vi "create func files.vi"(11 "path":path) -> (2 "funtions.c":string, 3 "funtions.h":string)   [LabVIEW 2010]
uses:
  read_excel_values.llb/GetXL_CellValues_2D_String.vi
panel:
  out "error out":errorcluster
  # "Type: U8, I8, U16, I16, U32, I32, U64, I64, FLOAT"
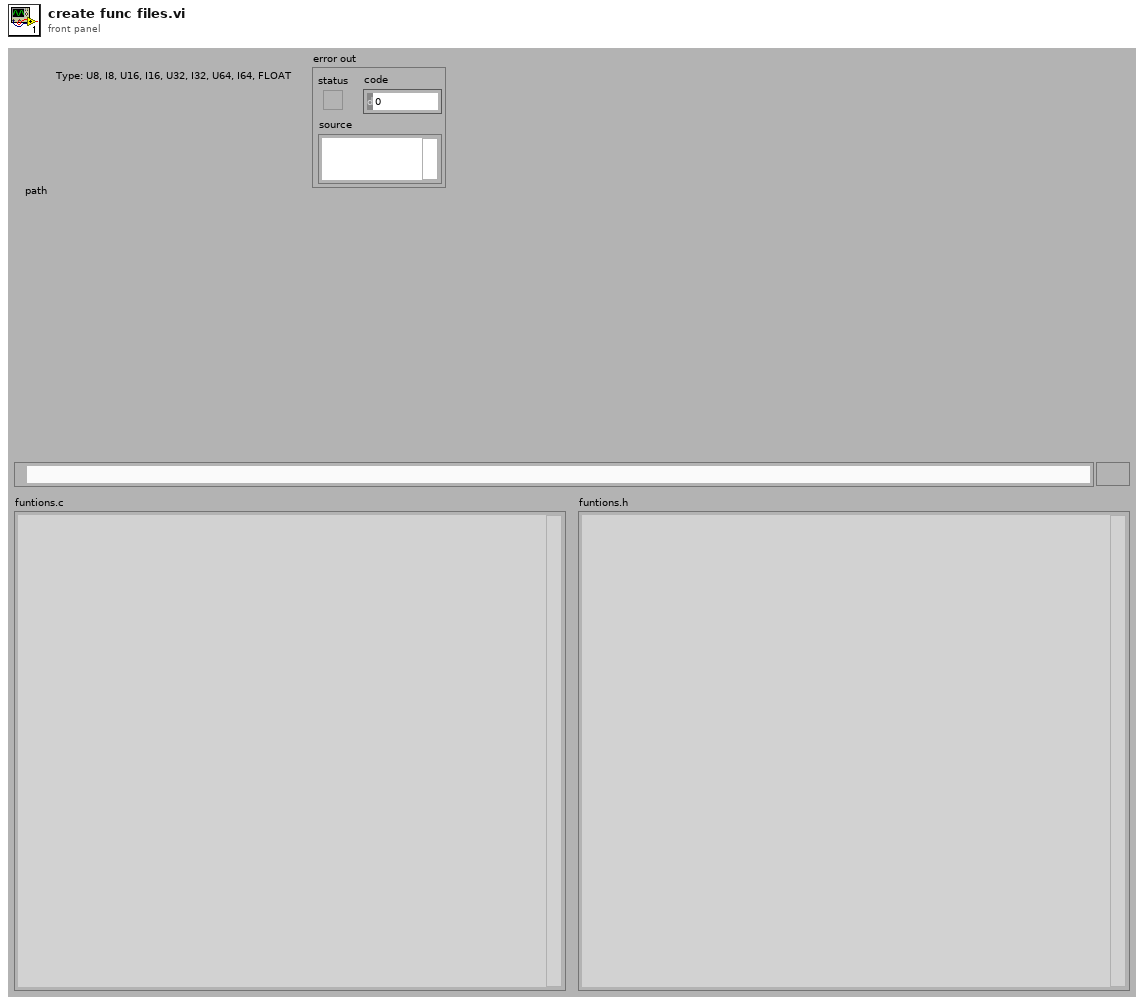
[diagram p1: front panel]
types:
  T1 = cluster{"Excel._Application":refnum<k7>, "Workbooks":refnum<k7>}
  T2 = cluster{"Excel._Application":refnum<k7>, "Workbooks":refnum<k7>, "Open":refnum<k7>}
  T3 = cluster{"Excel._Application":refnum<k7>, "Workbooks":refnum<k7>, "Open":refnum<k7>, "Worksheets":refnum<k7>, "Excel._Worksheet":refnum<k7>}
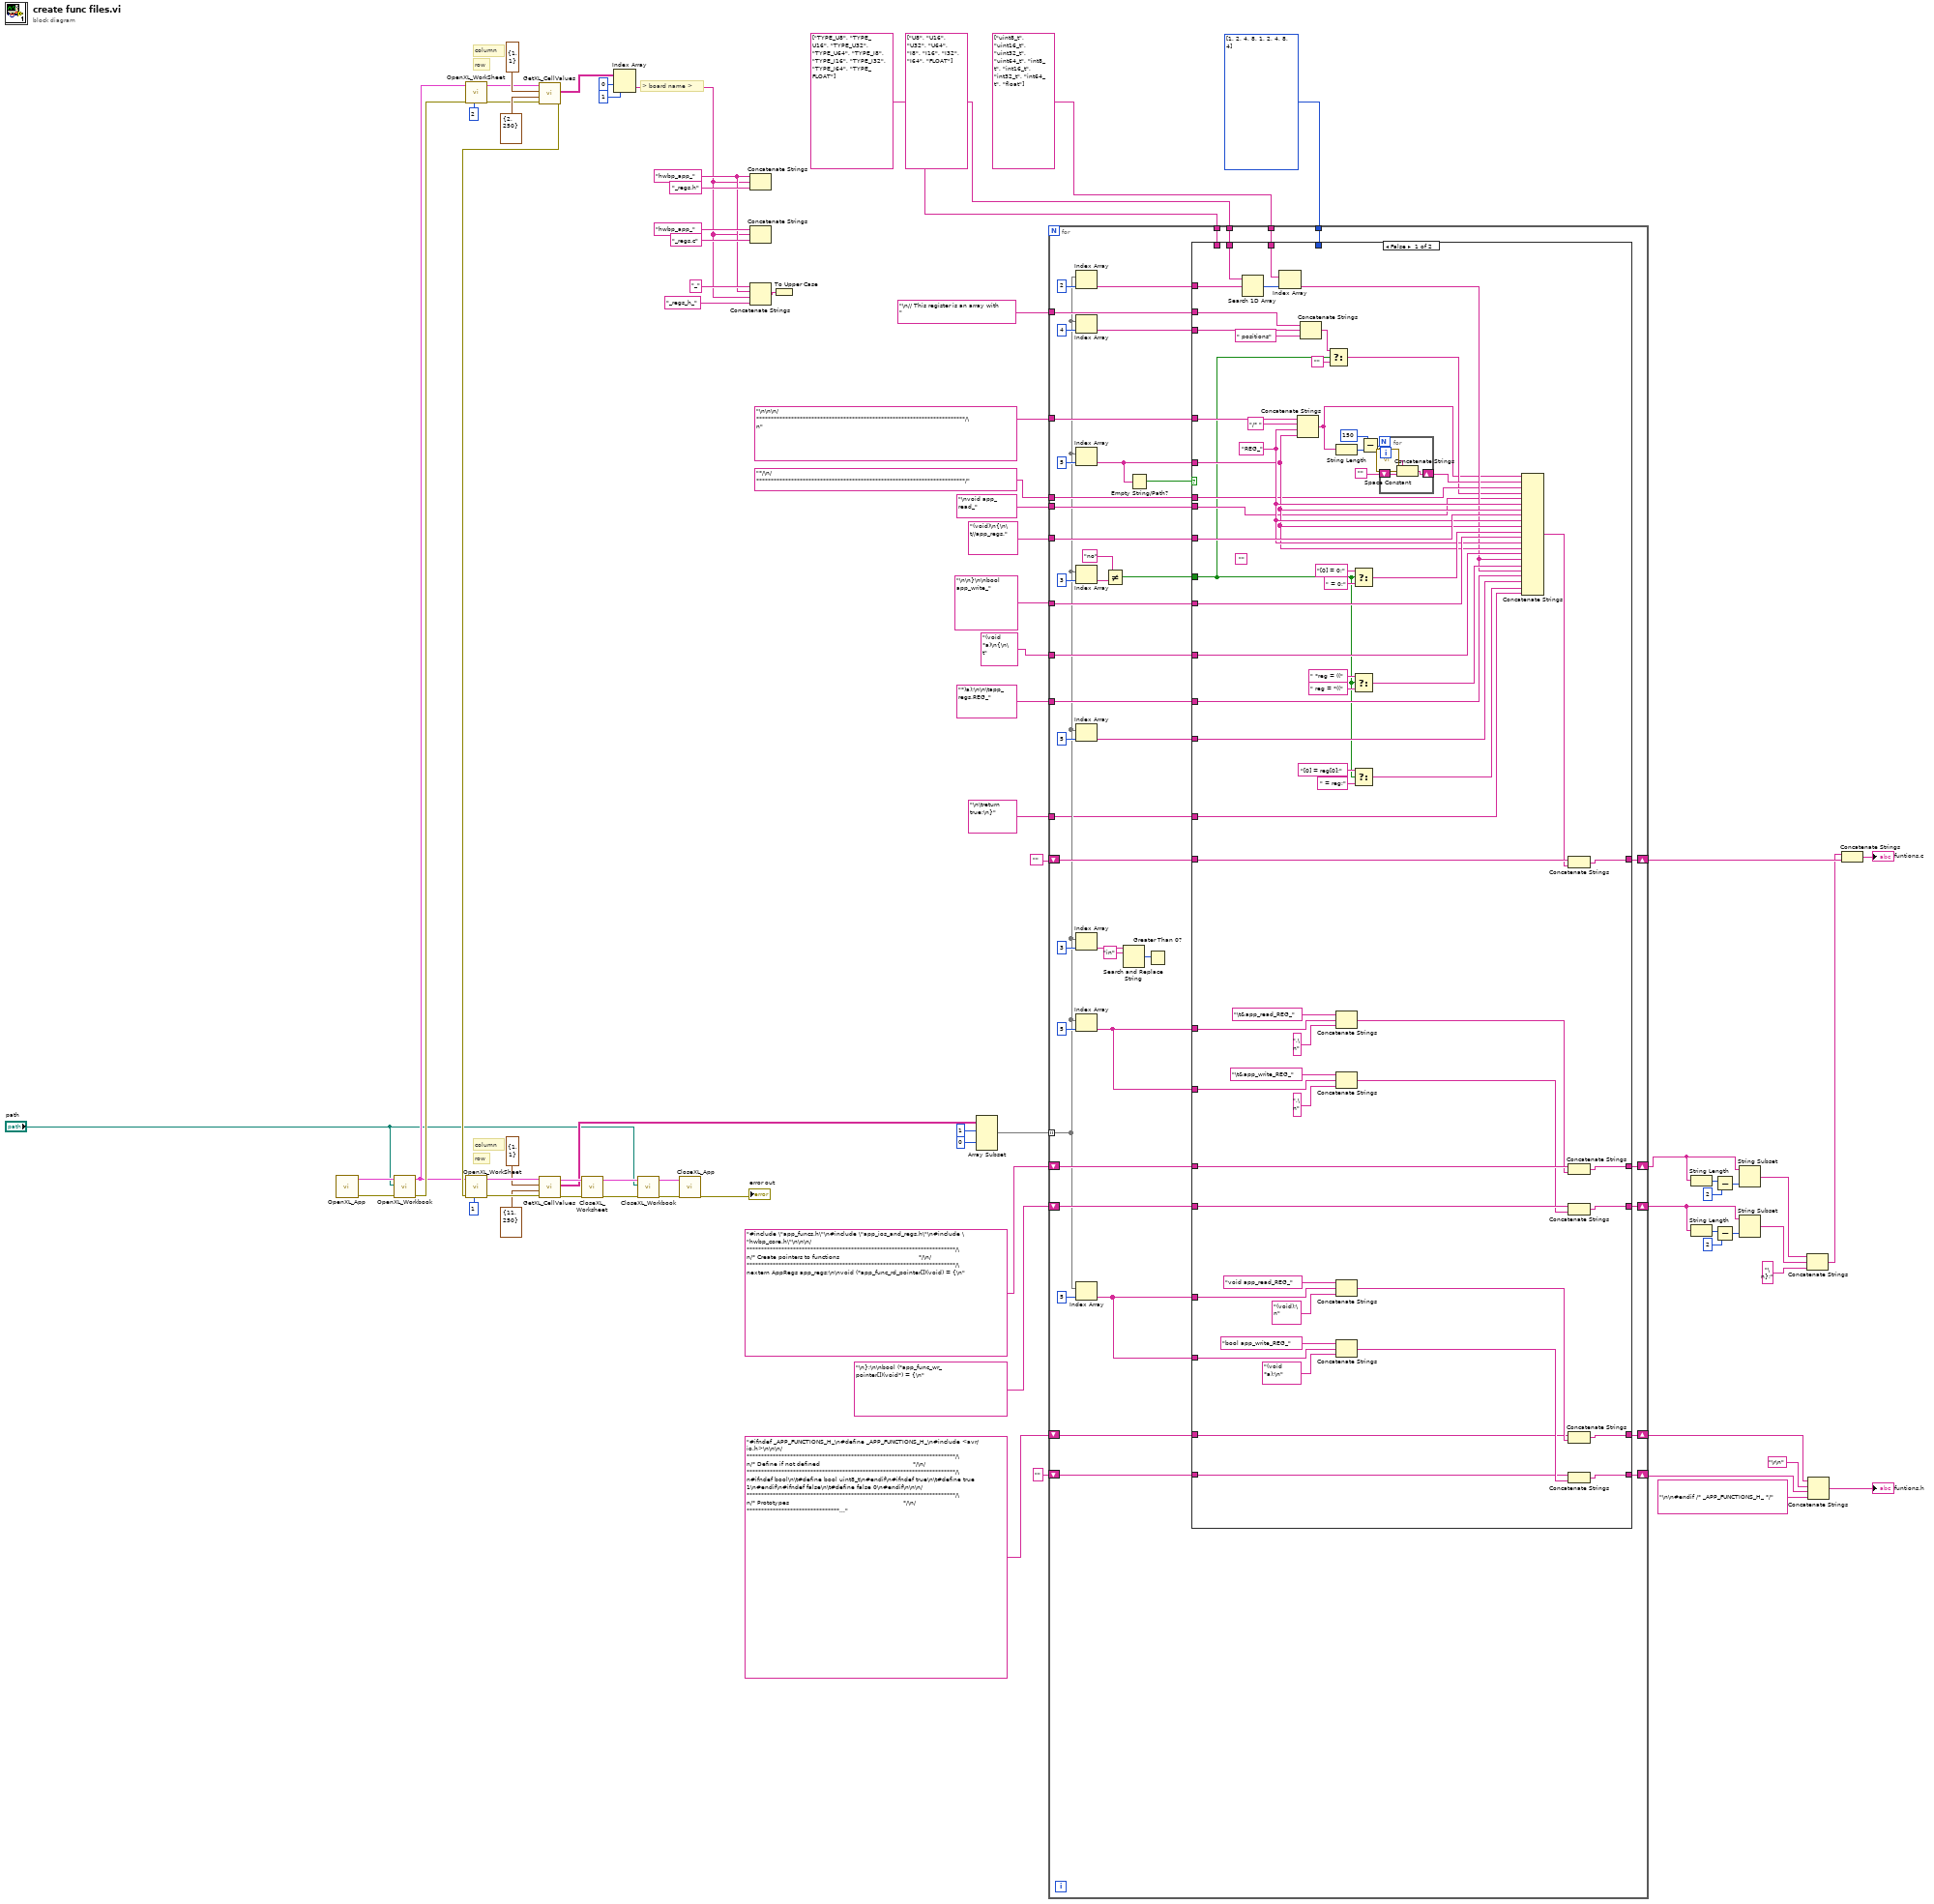
[diagram p0: block diagram]
diagram:
  w33 = "hwbp_app_" ("string")
  # "> board name >"
  # "row"
  # "column"
  # "row"
  # "column"
  n1 = call "OpenXL_App.vi"() -> ("error out"=w67:errorcluster, "Refnum Cluster"=w68:T1)  [unwired: 10 in]
  n2 = call "OpenXL_Workbook.vi"("error in"=w67, "path"="path", "Refnum Cluster In"=w68) -> ("error out"=w47:errorcluster, "Refnum Cluster Out"=w45:T2)  [unwired: 7 in]
  n3 = call "OpenXL_WorkSheet.vi"("Sheet"=2, "error in (no error)"=w47, "Refnum Cluster In"=w45) -> ("error out"=w49:errorcluster, "Refnum Cluster Out"=w48:T3)  [unwired: 7 in]
  n4 = call-poly "GetXL_CellValues.vi"("error in"=w49, "End"=cluster{"Column":i32, "Row":i32} {"Column"=2, "Row"=250}, "Start"=cluster{"Column":i32, "Row":i32} {"Column"=1, "Row"=1}, "Refnum Cluster In"=w48) -> ("error out"=w46:errorcluster, "data"=w42:string[][])  [unwired: 5 in, 1 out]
  n5 = call "OpenXL_WorkSheet.vi"("Sheet"=1, "error in (no error)"=w46, "Refnum Cluster In"=w45) -> ("error out"=w74:errorcluster, "Refnum Cluster Out"=w75:T3)  [unwired: 7 in]
  n6 = call-poly "GetXL_CellValues.vi"("error in"=w74, "End"=cluster{"Column":i32, "Row":i32} {"Column"=11, "Row"=250}, "Start"=cluster{"Column":i32, "Row":i32} {"Column"=1, "Row"=1}, "Refnum Cluster In"=w75) -> ("error out"=w65:errorcluster, "data"=w56:string[][], "Refnum Cluster Out"=w66:T3)  [unwired: 5 in]
  n7 = call "CloseXL_Worksheet.vi"("error in (no error)"=w65, "Refnum Cluster In"=w66) -> ("error out"=w63:errorcluster, "Refnum Cluster Out"=w64:T2)  [unwired: 8 in]
  n8 = Index Array(array=w42, index (row)=0, index (col)=1 ("disabled index (col)")) -> (element=w32:string)
  n9 = call "CloseXL_Workbook.vi"("error in (no error)"=w63, "path"="path", "Refnum Cluster In"=w64) -> ("error out"=w72:errorcluster, "Refnum Cluster Out"=w73:T1)  [unwired: 7 in]
  n10 = call "CloseXL_App.vi"("error in (no error)"=w72, "Refnum Cluster In"=w73) -> ("error out"=→"error out":errorcluster)  [unwired: 9 in]
  n11 = Concatenate Strings(w33, w32, "_regs.h" ("string")) -> ()  [unwired: 1 out]
  n12 = Concatenate Strings("hwbp_app_" ("string"), w32, "_regs.c" ("string")) -> ()  [unwired: 1 out]
  n13 = Concatenate Strings("_" ("string"), w33, w32, "_regs_h_" ("string")) -> (w35:string)
  n14 = To Upper Case(1:w35) -> ()  [unwired: 1 out]
  n15 = Array Subset(array=w56, index (row)=1 ("index"), index (col)=0 ("index")) -> (w53:string[][])  [unwired: 2 in]
  n16 = for {
    tunnel: w53 -> [w78] mode=indexing
    tunnel: string[] ["U8", "U16", "U32", "U64", "I8", "I16", "I32", "I64", "FLOAT"] -> [w120]
    tunnel: string[] ["uint8_t", "uint16_t", "uint32_t", "uint64_t", "int8_t", "int16_t", "int32_t", "int64_t", "float"] -> [w119]
    tunnel: i32[] [1, 2, 4, 8, 1, 2, 4, 8, 4] -> [w118]
    tunnel: string[] ["TYPE_U8", "TYPE_U16", "TYPE_U32", "TYPE_U64", "TYPE_I8", "TYPE_I16", "TYPE_I32", "TYPE_I64", "TYPE_FLOAT"] -> [w117]
    shift-right: [w114] -> w25
    shift-left: "" -> [w115]
    tunnel: "\n\n\n/************************************************************************/\n" ("x") -> [w110]
    tunnel: "*/\n/************************************************************************/" ("x") -> [w109]
    tunnel: "(void)\n{\n\t//app_regs." ("x") -> [w108]
    tunnel: "\n\n}\n\nbool app_write_" ("x") -> [w106]
    tunnel: "(void *a)\n{\n\t" ("x") -> [w105]
    tunnel: "*)a);\n\n\tapp_regs.REG_" ("string") -> [w102]
    tunnel: "\nvoid app_read_" ("x") -> [w93]
    tunnel: "\n// This register is an array with " ("string") -> [w92]
    shift-right: [w89] -> w11
    shift-left: "#include \"app_funcs.h\"\n#include \"app_ios_and_regs.h\"\n#include \"hwbp_core.h\"\n\n\n/************************************************************************/\n/* Create pointers to functions                                         */\n/************************************************************************/\nextern AppRegs app_regs;\n\nvoid (*app_func_rd_pointer[])(void) = {\n" ("string") -> [w88]
    shift-right: [w86] -> w19
    shift-left: "\n};\n\nbool (*app_func_wr_pointer[])(void*) = {\n" ("string") -> [w87]
    shift-right: [w82] -> w7
    shift-left: "#ifndef _APP_FUNCTIONS_H_\n#define _APP_FUNCTIONS_H_\n#include <avr/io.h>\n\n\n/************************************************************************/\n/* Define if not defined                                                */\n/************************************************************************/\n#ifndef bool\n\t#define bool uint8_t\n#endif\n#ifndef true\n\t#define true 1\n#endif\n#ifndef false\n\t#define false 0\n#endif\n\n\n/************************************************************************/\n/* Prototypes                                                           */\n/************************************************************************/\n" ("string") -> [w83]
    shift-right: [w85] -> w4
    shift-left: "" -> [w84]
    tunnel: "\n\treturn true;\n}" ("string") -> [w76]
    n17 = Index Array(array=w78, index=2) -> (element=w103:string)
    n18 = Index Array(array=w78, index=4) -> (element=w94:string)
    n19 = Index Array(array=w78, index=5) -> (element=w97:string)
    n20 = Index Array(array=w78, index=3) -> (element=w112:string)
    n21 = Index Array(array=w78, index=5) -> (element=w77:string)
    n22 = Index Array(array=w78, index=3) -> (element=w100:string)
    n23 = Index Array(array=w78, index=5) -> (element=w90:string)
    n24 = Index Array(array=w78, index=5) -> (element=w81:string)
    n25 = Not Equal?(x="no", y=w112) -> (x != y?=w107:bool)
    n26 = Search and Replace String(input string=w100, search string="in") -> (number of replacements=w98:i32)  [unwired: 6 in, 3 out]
    n27 = Empty String/Path?(string/path=w97) -> (empty?=w96:bool)
    n28 = Greater Than 0?(x=w98) -> ()  [unwired: 1 out]
    n29 = case shown="False" w96 {
      tunnel: w120 -> [w175 _]
      tunnel: w119 -> [w173 _]
      tunnel: w118 -> [_ _]
      tunnel: w117 -> [_ _]
      tunnel: w115 -> [w186 w194]
      tunnel: [w185 w194] -> w114
      tunnel: w110 -> [w171 _]
      tunnel: w109 -> [w155 _]
      tunnel: w108 -> [w169 _]
      tunnel: w107 -> [w123 _]
      tunnel: w106 -> [w167 _]
      tunnel: w105 -> [w164 _]
      tunnel: w103 -> [w174 _]
      tunnel: w102 -> [w161 _]
      tunnel: w97 -> [w165 _]
      tunnel: w94 -> [w160 _]
      tunnel: w93 -> [w154 _]
      tunnel: w92 -> [w152 _]
      tunnel: w90 -> [w149 _]
      tunnel: w90 -> [w145 _]
      tunnel: w88 -> [w143 w193]
      tunnel: [w144 w193] -> w89
      tunnel: w87 -> [w142 w192]
      tunnel: [w141 w192] -> w86
      tunnel: w81 -> [w128 _]
      tunnel: w81 -> [w132 _]
      tunnel: w83 -> [w134 w191]
      tunnel: [w133 w191] -> w82
      tunnel: w84 -> [w135 w190]
      tunnel: [w136 w190] -> w85
      tunnel: w77 -> [w126 _]
      tunnel: w76 -> [w121 _]
      frame False {
        (unwired) ""
        w166 = "REG_" ("string")
        n30 = Search 1D Array(1D array=w175, element=w174) -> (index of element=w176:i32)  [unwired: 1 in]
        n31 = Index Array(array=w173, index=w176) -> (element=w162:string)
        n32 = Concatenate Strings(w171, "/* " ("string"), w166, w165) -> (w151:string)
        n33 = Concatenate Strings(w152, w160, " positions" ("string")) -> (w158:string)
        n34 = Select(t=w158, s=w123, f="") -> (s? t:f=w153:string)
        n35 = String Length(string=w151) -> (length=w181:i32)
        n36 = Concatenate Strings("\t&app_read_REG_" ("string"), w149, ",\n" ("string")) -> (w140:string)
        n37 = Concatenate Strings("\t&app_write_REG_" ("string"), w145, ",\n" ("string")) -> (w139:string)
        n38 = Concatenate Strings("void app_read_REG_" ("string"), w128, "(void);\n" ("string")) -> (w137:string)
        n39 = Concatenate Strings("bool app_write_REG_" ("string"), w132, "(void *a);\n" ("string")) -> (w138:string)
        n40 = Select(t="[0] = 0;" ("string"), s=w123, f=" = 0;" ("string")) -> (s? t:f=w168:string)
        n41 = Select(t=" *reg = ((" ("string"), s=w123, f=" reg = *((" ("string")) -> (s? t:f=w163:string)
        n42 = Select(t="[0] = reg[0];" ("string"), s=w123, f=" = reg;" ("string")) -> (s? t:f=w122:string)
        n43 = Subtract(x=150, y=w181) -> (x-y=w183:i32)
        n44 = for {
          N: w183 -> [_]
          shift-right: [w187] -> w156
          shift-left: "" -> [w189]
          n45 = call <vilib>:"Space Constant.vi"() -> ("String"=w188:string)
          n46 = Concatenate Strings(w188, w189) -> (w187:string)
        }
        n47 = Concatenate Strings(w151, w156, w155, w153, w154, w166, w165, w169, w166, w165, w168, w167, w166, w165, w164, w162, w163, w162, w161, w126, w122, w121) -> (w172:string)
        n48 = Concatenate Strings(w186, w172) -> (w185:string)
        n49 = Concatenate Strings(w143, w140) -> (w144:string)
        n50 = Concatenate Strings(w142, w139) -> (w141:string)
        n51 = Concatenate Strings(w134, w137) -> (w133:string)
        n52 = Concatenate Strings(w135, w138) -> (w136:string)
      }
      frame True {
      }
    }
  }
  n53 = String Length(string=w11) -> (length=w12:i32)
  n54 = String Length(string=w19) -> (length=w22:i32)
  n55 = Subtract(x=w12, y=2 ("index")) -> (x-y=w14:i32)
  n56 = Subtract(x=w22, y=2 ("index")) -> (x-y=w20:i32)
  n57 = String Subset(string=w11, length (rest)=w14) -> (substring=w10:string)  [unwired: 1 in]
  n58 = String Subset(string=w19, length (rest)=w20) -> (substring=w15:string)  [unwired: 1 in]
  n59 = Concatenate Strings(w10, w15, "\n};" ("string")) -> (w9:string)
  n60 = Concatenate Strings(w7, "\r\n", w4, "\n\n#endif /* _APP_FUNCTIONS_H_ */" ("string")) -> (→"funtions.h":string)
  n61 = Concatenate Strings(w9, w25) -> (→"funtions.c":string)
